vi "metadata.get_request.vi"(8 "error in":errorcluster, 11 "channel in":refnum<class "Channel.lvclass">) -> (0 "error out":errorcluster, 3 "JSON Payload":string)   [LabVIEW 2020, in "Nominal Client.lvclass"]
uses:
  Nominal Client/Nominal Client.lvclass
  submodules/nominal-streaming-labview-ffi/lv_src/Channel/Channel.lvclass
  submodules/nominal-streaming-labview-ffi/lv_src/Channel/Channel.lvclass/Channel.ctl
  submodules/nominal-streaming-labview-ffi/lv_src/Stream/Stream.lvclass/Stream.ctl
  3536d236-6dd3-40ff-a9be-19a538437cb9.vi
  3b5d701c-bf98-49ac-9ba1-b856c1a1d350.vi
  submodules/nominal-streaming-labview-ffi/lv_src/Channel/name.get.vi
  submodules/nominal-streaming-labview-ffi/lv_src/Channel/stream.get.vi
  submodules/nominal-streaming-labview-ffi/lv_src/Stream/datasetRid.get.vi
  <vilib>/JDP Science/JSONtext/Variant to JSON Text.vi
  submodules/nominal-streaming-labview-ffi/lv_src/Stream/Stream.lvclass
  <vilib>/JDP Science/JSONtext/LVClass Serializer/JSONtext LVClass Serializer.lvclass
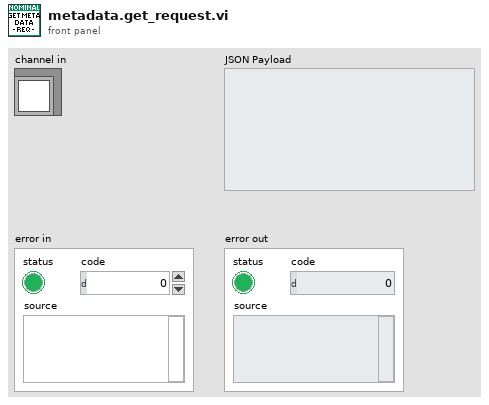
[diagram p1: front panel]
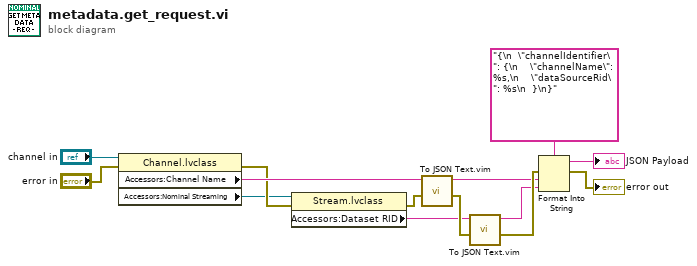
[diagram p0: block diagram]
diagram:
  n1 = property class="Channel.lvclass"(reference="channel in", error in="error in") -> (error out=w11:errorcluster, "Accessors:Channel Name"=w12:string, "Accessors:Nominal Streaming"=w2:refnum<class "Stream.lvclass">)  [unwired: 1 out]
  n2 = property class="Stream.lvclass"(reference=w2, error in=w11) -> (error out=w7:errorcluster, "Accessors:Dataset RID"=w1:string)  [unwired: 1 out]
  n3 = call "To JSON Text.vim"("error in (no error)"=w7, "Anything"=w12) -> ("error out"=w6:errorcluster, "<JSON>"=w4:string)  [unwired: 8 in]
  n4 = call "To JSON Text.vim"("error in (no error)"=w6, "Anything"=w1) -> ("error out"=w5:errorcluster, "<JSON>"=w3:string)  [unwired: 8 in]
  n5 = Format Into String(format string="{\n  \"channelIdentifier\": {\n    \"channelName\": %s,\n    \"dataSourceRid\": %s\n  }\n}", error in=w5, w4, w3) -> (resulting string=→"JSON Payload":string, error out=→"error out":errorcluster)  [unwired: 1 in]
